vi "ReadData.vi"(8 "error in":errorcluster, 11 "Module Config Selector":i16) -> (0 "error out":errorcluster, 1 "Number Of Pulses":u32, 2 "OversampleClk Ticks":u32, 3 "Data Array":sgl[](array[numeric]) format="%.2f")   [LabVIEW 2017, in "VDMS_VibAPI_8.lvlib"]
uses:
  <vilib>/addons/InsightCM/Devices/Shared/Cms/Fpga/AcquisitionFpgaTach/source/subVIs/VibAPI_8/VDMS_VibAPI_8.lvlib
  <vilib>/rvi/eio/common/nirviEmuTemplateMethod_errors.vi
  <vilib>/rvi/Memory/Memory_Emulation/nirvimemoryFastEmulation.vi
  <vilib>/rvi/Memory/Memory_Emulation/nirvimemoryEmulation.vi
  <vilib>/rvi/Emulation/niFpgaEmulationIsFPGAContextNoSignature.vi
  <vilib>/rvi/DataTransferAndStorage/Container/Common/niFpgaContainerGetUniqueNameForEmu.vi
  <vilib>/rvi/Emulation/niFpgaProcessEmulError.vi
  <vilib>/rvi/Emulation/niFpgaSctlEmulationGetInTimedLoop.vi
  <vilib>/rvi/errors/nirviReportUnexpectedCaseInternalError (U32).vi
  <vilib>/eio/EIONode/EIONode.xnode
  <vilib>/rvi/DataTransferAndStorage/Container/XNode/niFpgaContainer.xnode
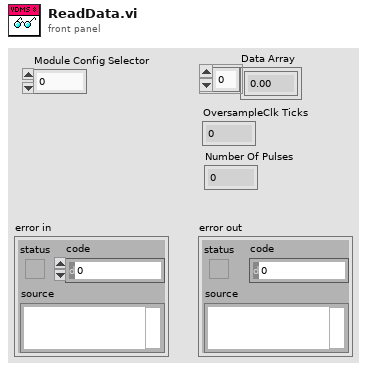
[diagram p1: front panel]
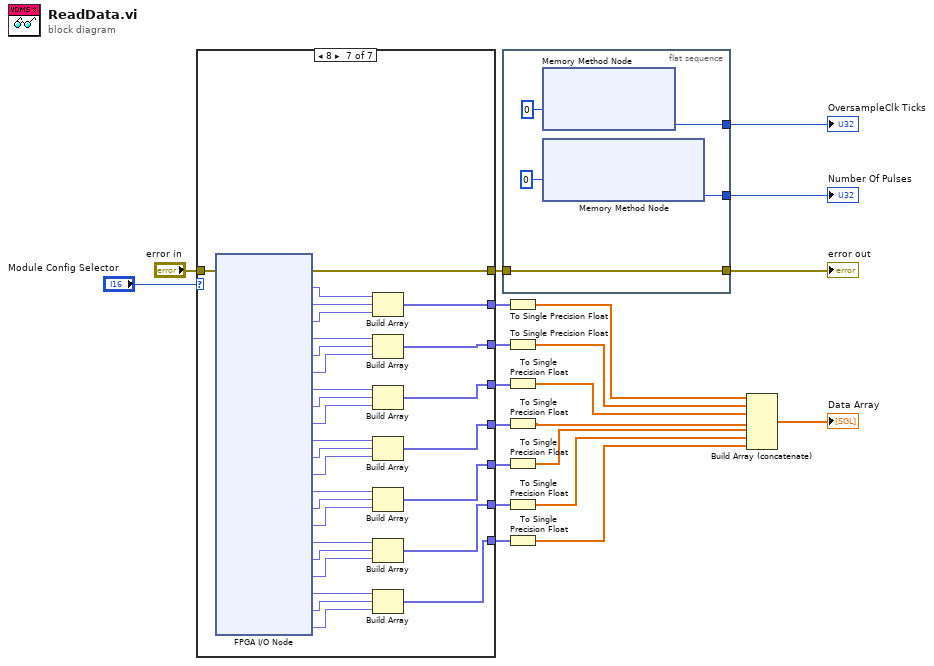
[diagram p0: block diagram]
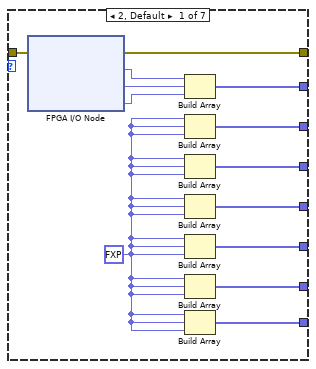
[diagram p2: hidden frame]
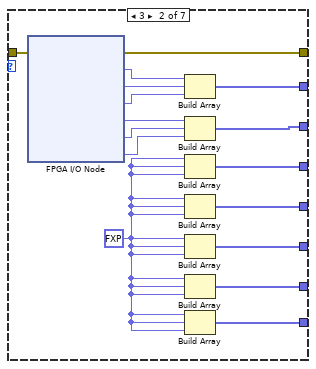
[diagram p3: hidden frame]
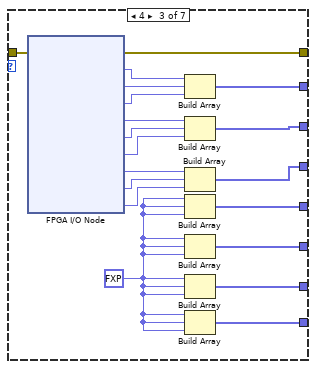
[diagram p4: hidden frame]
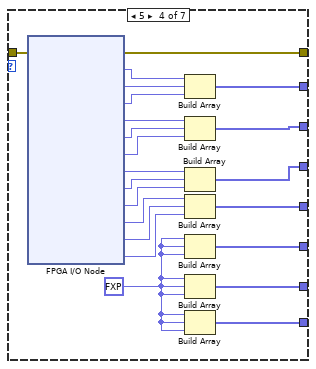
[diagram p5: hidden frame]
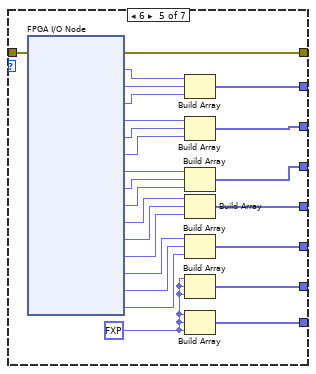
[diagram p6: hidden frame]
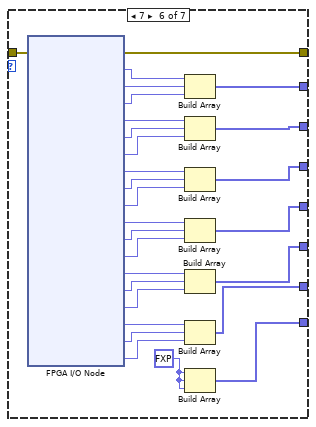
[diagram p7: hidden frame]
diagram:
  n1 = case shown="8" "Module Config Selector" {
    tunnel: "error in" -> [w34 w50 w69 w91 w116 w144 w174]
    tunnel: [w33 w49 w68 w90 w115 w143 w173] -> w19
    tunnel: [w32 w48 w67 w89 w114 w142 w172] -> w15
    tunnel: [w31 w47 w66 w88 w113 w141 w171] -> w13
    tunnel: [w30 w46 w65 w87 w112 w140 w170] -> w10
    tunnel: [w29 w45 w64 w86 w111 w139 w169] -> w8
    tunnel: [w28 w44 w63 w85 w110 w138 w168] -> w6
    tunnel: [w24 w37 w53 w84 w109 w137 w167] -> w4
    tunnel: [w22 w35 w51 w83 w108 w136 w166] -> w2
    frame 2, Default {
      w23 = fxp<+/-,24,7> 0.0 ("Mod1/AI2")
      n2 = xnode "FPGA I/O Node"("error in"=w34) -> ("error out"=w33:errorcluster, "Mod2/AI0"=w27:fxp<+/-,24,7>, "Mod2/AI1"=w26:fxp<+/-,24,7>, "Mod2/AI2"=w25:fxp<+/-,24,7>)  [unwired: 3 in, 3 out]
      n3 = Build Array(w27, w26, w25) -> (w32:fxp<+/-,24,7>[])
      n4 = Build Array(w23, w23, w23) -> (w31:fxp<+/-,24,7>[])
      n5 = Build Array(w23, w23, w23) -> (w30:fxp<+/-,24,7>[])
      n6 = Build Array(w23, w23, w23) -> (w29:fxp<+/-,24,7>[])
      n7 = Build Array(w23, w23, w23) -> (w28:fxp<+/-,24,7>[])
      n8 = Build Array(w23, w23, w23) -> (w24:fxp<+/-,24,7>[])
      n9 = Build Array(w23, w23, w23) -> (w22:fxp<+/-,24,7>[])
    }
    frame 3 {
      w36 = fxp<+/-,24,7> 0.0 ("Mod1/AI2")
      n10 = xnode "FPGA I/O Node"("error in"=w50) -> ("error out"=w49:errorcluster, "Mod2/AI0"=w43:fxp<+/-,24,7>, "Mod2/AI1"=w42:fxp<+/-,24,7>, "Mod2/AI2"=w41:fxp<+/-,24,7>, "Mod3/AI0"=w40:fxp<+/-,24,7>, "Mod3/AI1"=w39:fxp<+/-,24,7>, "Mod3/AI2"=w38:fxp<+/-,24,7>)  [unwired: 6 in, 6 out]
      n11 = Build Array(w43, w42, w41) -> (w48:fxp<+/-,24,7>[])
      n12 = Build Array(w40, w39, w38) -> (w47:fxp<+/-,24,7>[])
      n13 = Build Array(w36, w36, w36) -> (w46:fxp<+/-,24,7>[])
      n14 = Build Array(w36, w36, w36) -> (w45:fxp<+/-,24,7>[])
      n15 = Build Array(w36, w36, w36) -> (w44:fxp<+/-,24,7>[])
      n16 = Build Array(w36, w36, w36) -> (w37:fxp<+/-,24,7>[])
      n17 = Build Array(w36, w36, w36) -> (w35:fxp<+/-,24,7>[])
    }
    frame 4 {
      w52 = fxp<+/-,24,7> 0.0 ("Mod1/AI2")
      n18 = xnode "FPGA I/O Node"("error in"=w69) -> ("error out"=w68:errorcluster, "Mod2/AI0"=w62:fxp<+/-,24,7>, "Mod2/AI1"=w61:fxp<+/-,24,7>, "Mod2/AI2"=w60:fxp<+/-,24,7>, "Mod3/AI0"=w59:fxp<+/-,24,7>, "Mod3/AI1"=w58:fxp<+/-,24,7>, "Mod3/AI2"=w57:fxp<+/-,24,7>, "Mod4/AI0"=w56:fxp<+/-,24,7>, "Mod4/AI1"=w55:fxp<+/-,24,7>, "Mod4/AI2"=w54:fxp<+/-,24,7>)  [unwired: 9 in, 9 out]
      n19 = Build Array(w62, w61, w60) -> (w67:fxp<+/-,24,7>[])
      n20 = Build Array(w59, w58, w57) -> (w66:fxp<+/-,24,7>[])
      n21 = Build Array(w56, w55, w54) -> (w65:fxp<+/-,24,7>[])
      n22 = Build Array(w52, w52, w52) -> (w64:fxp<+/-,24,7>[])
      n23 = Build Array(w52, w52, w52) -> (w63:fxp<+/-,24,7>[])
      n24 = Build Array(w52, w52, w52) -> (w53:fxp<+/-,24,7>[])
      n25 = Build Array(w52, w52, w52) -> (w51:fxp<+/-,24,7>[])
    }
    frame 5 {
      w70 = fxp<+/-,24,7> 0.0 ("Mod1/AI2")
      n26 = xnode "FPGA I/O Node"("error in"=w91) -> ("error out"=w90:errorcluster, "Mod2/AI0"=w82:fxp<+/-,24,7>, "Mod2/AI1"=w81:fxp<+/-,24,7>, "Mod2/AI2"=w80:fxp<+/-,24,7>, "Mod3/AI0"=w79:fxp<+/-,24,7>, "Mod3/AI1"=w78:fxp<+/-,24,7>, "Mod3/AI2"=w77:fxp<+/-,24,7>, "Mod4/AI0"=w76:fxp<+/-,24,7>, "Mod4/AI1"=w75:fxp<+/-,24,7>, "Mod4/AI2"=w74:fxp<+/-,24,7>, "Mod5/AI0"=w73:fxp<+/-,24,7>, "Mod5/AI1"=w72:fxp<+/-,24,7>, "Mod5/AI2"=w71:fxp<+/-,24,7>)  [unwired: 12 in, 12 out]
      n27 = Build Array(w82, w81, w80) -> (w89:fxp<+/-,24,7>[])
      n28 = Build Array(w79, w78, w77) -> (w88:fxp<+/-,24,7>[])
      n29 = Build Array(w76, w75, w74) -> (w87:fxp<+/-,24,7>[])
      n30 = Build Array(w73, w72, w71) -> (w86:fxp<+/-,24,7>[])
      n31 = Build Array(w70, w70, w70) -> (w85:fxp<+/-,24,7>[])
      n32 = Build Array(w70, w70, w70) -> (w84:fxp<+/-,24,7>[])
      n33 = Build Array(w70, w70, w70) -> (w83:fxp<+/-,24,7>[])
    }
    frame 6 {
      w92 = fxp<+/-,24,7> 0.0 ("Mod1/AI2")
      n34 = xnode "FPGA I/O Node"("error in"=w116) -> ("error out"=w115:errorcluster, "Mod2/AI0"=w107:fxp<+/-,24,7>, "Mod2/AI1"=w106:fxp<+/-,24,7>, "Mod2/AI2"=w105:fxp<+/-,24,7>, "Mod3/AI0"=w104:fxp<+/-,24,7>, "Mod3/AI1"=w103:fxp<+/-,24,7>, "Mod3/AI2"=w102:fxp<+/-,24,7>, "Mod4/AI0"=w101:fxp<+/-,24,7>, "Mod4/AI1"=w100:fxp<+/-,24,7>, "Mod4/AI2"=w99:fxp<+/-,24,7>, "Mod5/AI0"=w98:fxp<+/-,24,7>, "Mod5/AI1"=w97:fxp<+/-,24,7>, "Mod5/AI2"=w96:fxp<+/-,24,7>, "Mod6/AI0"=w95:fxp<+/-,24,7>, "Mod6/AI1"=w94:fxp<+/-,24,7>, "Mod6/AI2"=w93:fxp<+/-,24,7>)  [unwired: 15 in, 15 out]
      n35 = Build Array(w107, w106, w105) -> (w114:fxp<+/-,24,7>[])
      n36 = Build Array(w104, w103, w102) -> (w113:fxp<+/-,24,7>[])
      n37 = Build Array(w101, w100, w99) -> (w112:fxp<+/-,24,7>[])
      n38 = Build Array(w98, w97, w96) -> (w111:fxp<+/-,24,7>[])
      n39 = Build Array(w95, w94, w93) -> (w110:fxp<+/-,24,7>[])
      n40 = Build Array(w92, w92, w92) -> (w109:fxp<+/-,24,7>[])
      n41 = Build Array(w92, w92, w92) -> (w108:fxp<+/-,24,7>[])
    }
    frame 7 {
      w117 = fxp<+/-,24,7> 0.0 ("Mod1/AI2")
      n42 = xnode "FPGA I/O Node"("error in"=w144) -> ("error out"=w143:errorcluster, "Mod2/AI0"=w121:fxp<+/-,24,7>, "Mod2/AI1"=w122:fxp<+/-,24,7>, "Mod2/AI2"=w123:fxp<+/-,24,7>, "Mod3/AI0"=w124:fxp<+/-,24,7>, "Mod3/AI1"=w125:fxp<+/-,24,7>, "Mod3/AI2"=w126:fxp<+/-,24,7>, "Mod4/AI0"=w127:fxp<+/-,24,7>, "Mod4/AI1"=w128:fxp<+/-,24,7>, "Mod4/AI2"=w129:fxp<+/-,24,7>, "Mod5/AI0"=w130:fxp<+/-,24,7>, "Mod5/AI1"=w131:fxp<+/-,24,7>, "Mod5/AI2"=w132:fxp<+/-,24,7>, "Mod6/AI0"=w133:fxp<+/-,24,7>, "Mod6/AI1"=w134:fxp<+/-,24,7>, "Mod6/AI2"=w135:fxp<+/-,24,7>, "Mod7/AI0"=w120:fxp<+/-,24,7>, "Mod7/AI1"=w119:fxp<+/-,24,7>, "Mod7/AI2"=w118:fxp<+/-,24,7>)  [unwired: 18 in, 18 out]
      n43 = Build Array(w121, w122, w123) -> (w142:fxp<+/-,24,7>[])
      n44 = Build Array(w124, w125, w126) -> (w141:fxp<+/-,24,7>[])
      n45 = Build Array(w127, w128, w129) -> (w140:fxp<+/-,24,7>[])
      n46 = Build Array(w130, w131, w132) -> (w139:fxp<+/-,24,7>[])
      n47 = Build Array(w133, w134, w135) -> (w138:fxp<+/-,24,7>[])
      n48 = Build Array(w120, w119, w118) -> (w137:fxp<+/-,24,7>[])
      n49 = Build Array(w117, w117, w117) -> (w136:fxp<+/-,24,7>[])
    }
    frame 8 {
      n50 = xnode "FPGA I/O Node"("error in"=w174) -> ("error out"=w173:errorcluster, "Mod2/AI0"=w151:fxp<+/-,24,7>, "Mod2/AI1"=w152:fxp<+/-,24,7>, "Mod2/AI2"=w153:fxp<+/-,24,7>, "Mod3/AI0"=w154:fxp<+/-,24,7>, "Mod3/AI1"=w155:fxp<+/-,24,7>, "Mod3/AI2"=w156:fxp<+/-,24,7>, "Mod4/AI0"=w157:fxp<+/-,24,7>, "Mod4/AI1"=w158:fxp<+/-,24,7>, "Mod4/AI2"=w159:fxp<+/-,24,7>, "Mod5/AI0"=w160:fxp<+/-,24,7>, "Mod5/AI1"=w161:fxp<+/-,24,7>, "Mod5/AI2"=w162:fxp<+/-,24,7>, "Mod6/AI0"=w163:fxp<+/-,24,7>, "Mod6/AI1"=w164:fxp<+/-,24,7>, "Mod6/AI2"=w165:fxp<+/-,24,7>, "Mod7/AI0"=w150:fxp<+/-,24,7>, "Mod7/AI1"=w149:fxp<+/-,24,7>, "Mod7/AI2"=w148:fxp<+/-,24,7>, "Mod8/AI0"=w147:fxp<+/-,24,7>, "Mod8/AI1"=w146:fxp<+/-,24,7>, "Mod8/AI2"=w145:fxp<+/-,24,7>)  [unwired: 21 in, 21 out]
      n51 = Build Array(w151, w152, w153) -> (w172:fxp<+/-,24,7>[])
      n52 = Build Array(w154, w155, w156) -> (w171:fxp<+/-,24,7>[])
      n53 = Build Array(w157, w158, w159) -> (w170:fxp<+/-,24,7>[])
      n54 = Build Array(w160, w161, w162) -> (w169:fxp<+/-,24,7>[])
      n55 = Build Array(w163, w164, w165) -> (w168:fxp<+/-,24,7>[])
      n56 = Build Array(w150, w149, w148) -> (w167:fxp<+/-,24,7>[])
      n57 = Build Array(w147, w146, w145) -> (w166:fxp<+/-,24,7>[])
    }
  }
  n58 = flat-sequence {
    tunnel: w19 -> [w179]
    tunnel: [w179] -> w18
    tunnel: [w178] -> w17
    tunnel: [w175] -> w16
    frame #0 {
      n59 = xnode ("Memory Method Node")("Address"=u32 0) -> ("Data"=w178:u32)  [unwired: 1 in, 1 out]
      n60 = xnode ("Memory Method Node")("Address"=u32 0) -> ("Data"=w175:u32)  [unwired: 1 in, 1 out]
    }
  }
  n61 = To Single Precision Float(number=w15) -> (single precision float=w14:sgl[])
  n62 = To Single Precision Float(number=w13) -> (single precision float=w12:sgl[])
  n63 = To Single Precision Float(number=w10) -> (single precision float=w9:sgl[])
  n64 = To Single Precision Float(number=w8) -> (single precision float=w7:sgl[])
  n65 = To Single Precision Float(number=w6) -> (single precision float=w5:sgl[])
  n66 = To Single Precision Float(number=w4) -> (single precision float=w3:sgl[])
  n67 = To Single Precision Float(number=w2) -> (single precision float=w1:sgl[])
  n68 = Build Array (concatenate)(w14, w12, w9, w7, w5, w3, w1) -> (→"Data Array":sgl[])
  "error out" <- w18
  "OversampleClk Ticks" <- w17
  "Number Of Pulses" <- w16
